vi "set_chart_x_range.vi"(9 "ref_chart":refnum<vi>, 11 "ref_x_range":refnum<vi>) -> ()   [LabVIEW 2019]
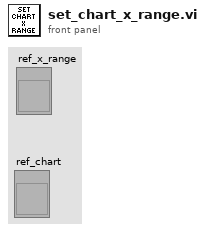
[diagram p1: front panel]
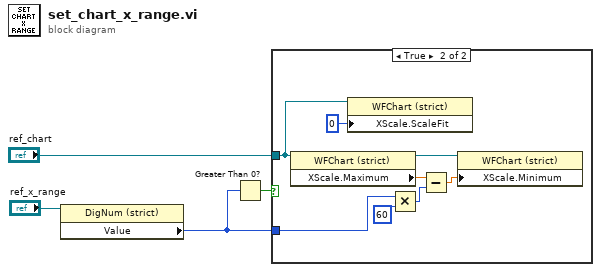
[diagram p0: block diagram]
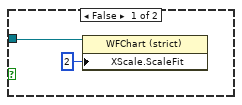
[diagram p2: hidden frame]
diagram:
  n1 = property class="DigNum (strict)"(reference="ref_x_range") -> ("Value"=w4:u32)  [unwired: 1 in, 2 out]
  n2 = Greater Than 0?(x=w4) -> (x > 0?=w3:bool)
  n3 = case shown="True" w3 {
    tunnel: "ref_chart" -> [w6 w7]
    tunnel: w4 -> [_ w10]
    frame False {
      n4 = property class="WFChart (strict)"(reference=w6, "XScale.ScaleFit"=u8 2 ("X Scale.Scale Fit")) -> ()  [unwired: 1 in, 2 out]
    }
    frame True {
      n5 = property class="WFChart (strict)"(reference=w7) -> (reference out=w14:refnum<vi>, "XScale.Maximum"=w13:dbl)  [unwired: 1 in, 1 out]
      n6 = property class="WFChart (strict)"(reference=w7, "XScale.ScaleFit"=u8 0 ("X Scale.Scale Fit")) -> ()  [unwired: 1 in, 2 out]
      n7 = Multiply(x=w10, y=60) -> (x*y=w11:u32)
      n8 = Subtract(x=w13, y=w11) -> (x-y=w12:dbl)
      n9 = property class="WFChart (strict)"(reference=w14, "XScale.Minimum"=w12) -> ()  [unwired: 1 in, 2 out]
    }
  }
